vi "AB_API Apply Setting.vi"(8 "error in (no error)":errorcluster, 10 "Settings":T1, 11 "Source in":refnum<class "AB_Source.lvclass">) -> (0 "error out":errorcluster, 3 "Source out":refnum<class "AB_Source.lvclass">)   [LabVIEW 2020]
uses:
  <vilib>/AppBuilder/AB_Classes/Source/AB_Source.lvclass
  <vilib>/AppBuilder/AB_API/common/AB_API Apply Setting Type.ctl
  <vilib>/AppBuilder/AB_Classes/Source/Container/AB_Source_Container.lvclass
  e:/builds/penguin/labview/branches/2020/dev/dist/vi.lib/AppBuilder/AB_Classes/Source/AB_Source.lvclass
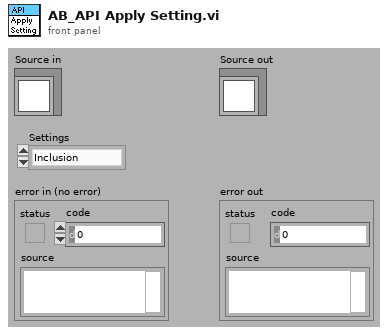
[diagram p1: front panel]
types:
  T1 = typedef "AB_API Apply Setting Type.ctl" = enum16{"Inclusion", "Destination", "Properties", "Password", "Prefix", "SaveSettings"}
  T2 = typedef "AB_Source_Container.ctl" = cluster{"applyInclusion":bool, "applyDestination":bool, "applyProperties":bool, "applyPassword":bool, "applyPrefix":bool, "applySaveSetttings":bool, "dependentDestinationIndex":i32}
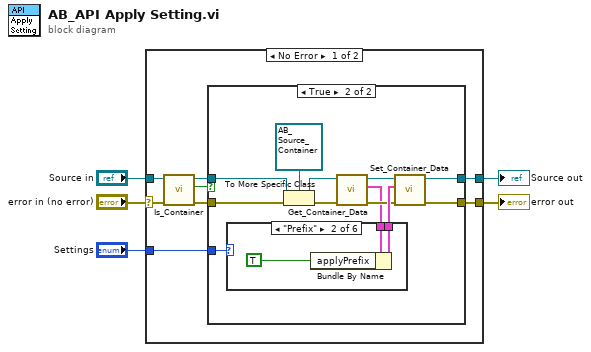
[diagram p0: block diagram]
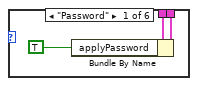
[diagram p3: hidden frame]
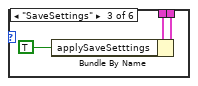
[diagram p4: hidden frame]
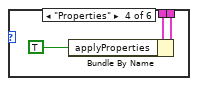
[diagram p5: hidden frame]
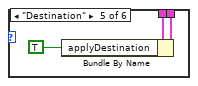
[diagram p6: hidden frame]
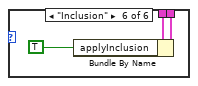
[diagram p7: hidden frame]
diagram:
  n1 = case shown="No Error" "error in (no error)" {
    selector: "error in (no error)" -> [w7 w46]
    tunnel: [w12 w46] -> w5
    tunnel: [w10 w47] -> w4
    tunnel: "Source in" -> [w8 w47]
    tunnel: "Settings" -> [w6 _]
    frame No Error {
      n2 = call-dynamic "Is_Container.vi"("error in (no error)"=w7, "AB_Source in"=w8) -> ("error out"=w11:errorcluster, "container"=w13:bool, "AB_Source out"=w9:refnum<class "AB_Source.lvclass">)  [unwired: 7 in]
      n3 = case shown="True" w13 {
        tunnel: w9 -> [w15 w21]
        tunnel: [w15 w20] -> w10
        tunnel: w11 -> [w14 w19]
        tunnel: [w14 w18] -> w12
        tunnel: w6 -> [_ w17]
        frame False {
        }
        frame True {
          n4 = To More Specific Class(target class=refnum<class "AB_Source_Container.lvclass"> refnum ("nullClass"), reference=w21, error in=w19) -> (specific class reference=w22:refnum<class "AB_Source_Container.lvclass">, error out=w24:errorcluster)
          n5 = call <vilib>:"Get_Container_Data.vi"("error in (no error)"=w24, "Class in"=w22) -> ("error out"=w23:errorcluster, "data"=w16:T2, "Class out"=w26:refnum<class "AB_Source_Container.lvclass">)  [unwired: 7 in]
          n6 = case shown="\"Prefix\"" w17 {
            tunnel: w16 -> [w29 w32 w35 w38 w41 w44]
            tunnel: [w28 w31 w34 w37 w40 w43] -> w25
            frame "Password" {
              n7 = Bundle By Name(cluster=w29, "applyPassword"=TRUE) -> (w28:T2)
            }
            frame "Prefix" {
              n8 = Bundle By Name(cluster=w32, "applyPrefix"=TRUE ("applyPassword")) -> (w31:T2)
            }
            frame "SaveSettings" {
              n9 = Bundle By Name(cluster=w35, "applySaveSetttings"=TRUE ("applyPassword")) -> (w34:T2)
            }
            frame "Properties" {
              n10 = Bundle By Name(cluster=w38, "applyProperties"=TRUE ("applyPassword")) -> (w37:T2)
            }
            frame "Destination" {
              n11 = Bundle By Name(cluster=w41, "applyDestination"=TRUE ("applyPassword")) -> (w40:T2)
            }
            frame "Inclusion" {
              n12 = Bundle By Name(cluster=w44, "applyInclusion"=TRUE ("applyPassword")) -> (w43:T2)
            }
          }
          n13 = call <vilib>:"Set_Container_Data.vi"("error in (no error)"=w23, "data"=w25, "Class in"=w26) -> ("error out"=w18:errorcluster, "Class out"=w20:refnum<class "AB_Source_Container.lvclass">)  [unwired: 7 in]
        }
      }
    }
    frame Error {
    }
  }
  "error out" <- w5
  "Source out" <- w4
